vi "new Wall.vi"(8 "error in (no error)":errorcluster) -> (0 "error out":errorcluster, 3 "Wall* out":refnum<data-value>)   [LabVIEW 2016, in "Wall.lvclass"]
uses:
  Wall.lvclass
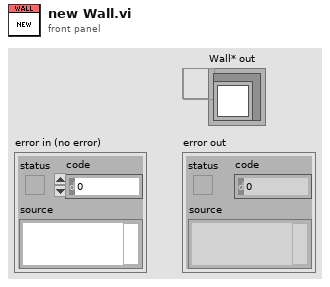
[diagram p1: front panel]
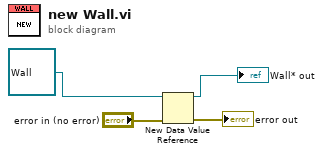
[diagram p0: block diagram]
diagram:
  n1 = New Data Value Reference(data value=refnum<class "Wall.lvclass"> refnum ("Wall in"), error in="error in (no error)") -> (data value reference=→"Wall* out":refnum<data-value>, error out=→"error out":errorcluster)
